vi "Create Execution Unit.vi"(8 "error in":errorcluster, 10 "Item Ref":T2=18446744073709551615 format="%.0x", 11 "Execution Unit Factory Implementation in":refnum<class "Execution Unit Factory.lvclass">) -> (0 "error out":errorcluster, 1 "Asynchronous Execution Units":T1[](array[typedef]) {"ReadWrite Channels" format="%.0x"; "Outgoing Channels" format="%.0x"; "Incoming Channels" format="%.0x"}, 2 "Inline Execution Units":T1[](array[typedef]) {"ReadWrite Channels" format="%.0x"; "Outgoing Channels" format="%.0x"; "Incoming Channels" format="%.0x"}, 3 "Execution Unit Factory Implementation out":refnum<class "Execution Unit Factory.lvclass">)   [LabVIEW 2020, in "Ballard ARINC 429 Engine.lvlib" / "Implementation.lvlib" / "Execution Unit Factory.lvclass"]
uses:
  Execution Unit Factory.lvclass
  <vilib>/NI VeriStand/Custom Device API/Custom Device Item Ref.ctl
  Interfaces/Controls/Execution Unit Information.ctl
  Interfaces/Execution Unit/Execution Unit.lvclass
  Rx Execution Unit/Rx Execution Unit.lvclass
  C:/Users/Administrator/Desktop/GIT/niveristand-ballard-arinc429-custom-device/Source/Custom Device Support/Engine/Interfaces/Execution Unit/Execution Unit.lvclass
  Tx Acyclic Labels Execution Unit/Tx Acyclic Labels Execution Unit.lvclass
  Tx Scheduled Labels Execution Unit/Tx Scheduled Labels Execution Unit.lvclass
  Execution Unit Factory.lvclass/Execution Unit Factory.ctl
  <vilib>/NI VeriStand/Custom Device API/Custom Device API.lvlib
  Interfaces/Interfaces.lvlib
  System Explorer/Implementation/Implementation.lvlib
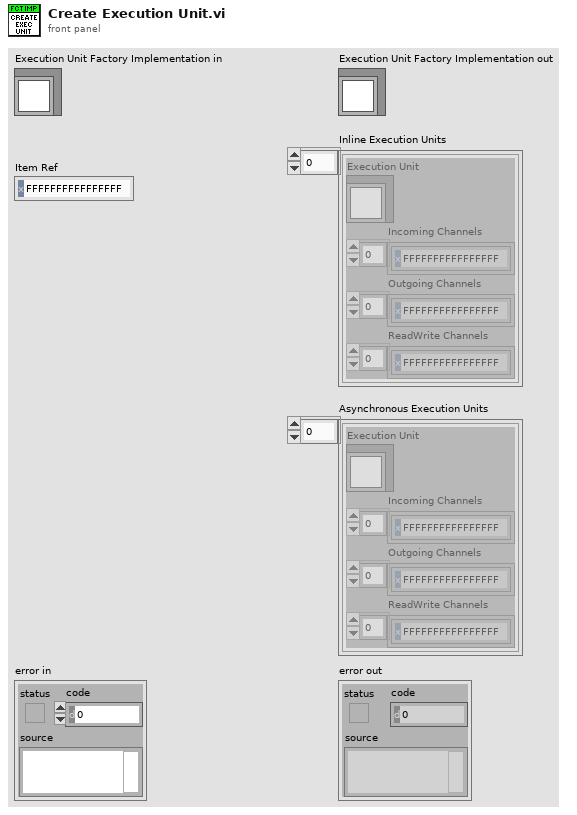
[diagram p1: front panel]
types:
  T1 = typedef "Ballard ARINC 429 Engine.lvlib/Interfaces.lvlib/Execution Unit Information.ctl" = cluster{"Execution Unit":refnum<class "Execution Unit.lvclass">, "Incoming Channels":T2[], "Outgoing Channels":T2[], "ReadWrite Channels":T2[]}
  T2 = typedef "Custom Device API.lvlib/Custom Device Item Ref.ctl" = u64
  T3 = typedef "Custom Device API.lvlib/Data Reference.ctl" = i32
  T4 = cluster{"receiving":T3, "specific errors":cluster{"gap":T3, "parity":T3, "long word ":T3, "bit timing":T3, "timeout":T3}}
  T5 = typedef "RT Hardware Channel Settings.ctl" = cluster{"channel #":u16, "channel handle":u64, "labels settings for RT":T6[]}
  T6 = typedef "RT Label Settings.ctl" = cluster{"Name":string, "xmlName":string, "label":T7, "transfer period":u32, "SDI_Enabled":bool, "SDI":u8, "parameter driver data":T8, "transfer type":T11, "has timestamp?":bool, "Label Disable/Trigger Channel Reference":T2, "Message Handle":u64, "Initialized?":bool, "Word Initial Raw Value":u32, "Label Timestamp Channel Data Reference":T3, "disabled":bool}
  T7 = typedef "Label.ctl" = u8
  T8 = typedef "RT Parameters.ctl" = cluster{"parameter definitions":T9[], "Tx parameter refs":T2[]}
  T9 = typedef "Parameter Definition.ctl" = cluster{"start index":i32, "size":i32, "encoding":T10, "signed":bool, "scale multiplier":dbl, "scale offset":dbl}
  T10 = typedef "Encoding and Decoding.lvlib/Encoding.ctl" = enum16{"BNR", "BCD", "Discrete"}
  T11 = typedef "Transfer Type.ctl" = enum16{"Scheduled", "Acyclic", "Block", "Strobe"}
  T12 = typedef "Custom Device API.lvlib/Custom Device Item Info.ctl" = cluster{"Name":string, "Is Channel":bool, "GUID":string, "Is Waveform":bool}
  T13 = cluster{"transfer type":T11, "Name":string, "hardware channel data":T5[], "Outgoing Channels":T2[], "ReadWrite Channels":T2[]}[]
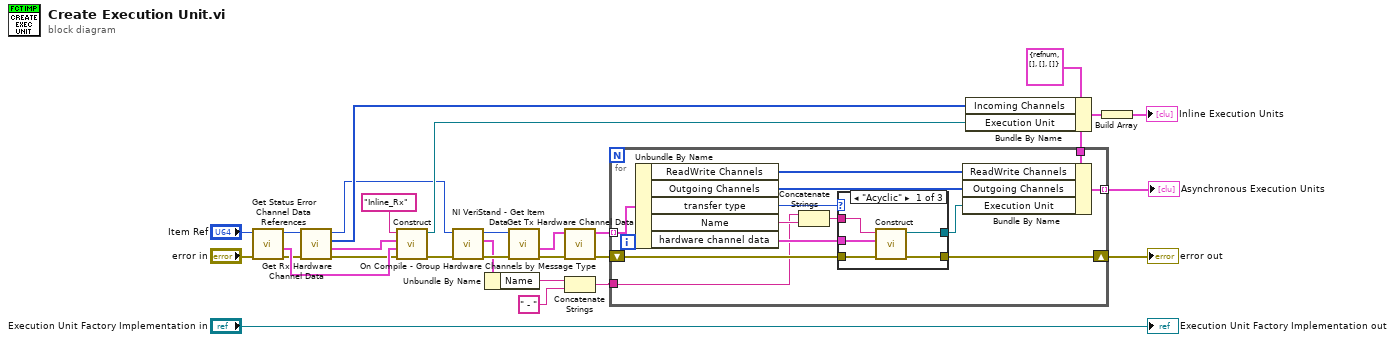
[diagram p0: block diagram]
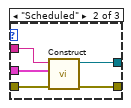
[diagram p2: hidden frame]
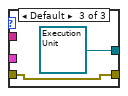
[diagram p3: hidden frame]
diagram:
  w10 = T1 {"Execution Unit"=refnum, "Incoming Channels"=[], "Outgoing Channels"=[], "ReadWrite Channels"=[]} ("Execution Unit Information")
  n1 = call "Get Status Error Channel Data References.vi"("error in"="error in", "custom device ref in"="Item Ref") -> ("error out"=w16:errorcluster, "status channel data references"=w20:T4, "custom device ref out"=w17:T2)  [unwired: 7 in]
  n2 = call "Get Rx Hardware Channel Data.vi"("error in"=w16, "custom device ref in"=w17) -> ("error out"=w15:errorcluster, "Rx hardware channel data"=w21:T5[], "incoming channels"=w25:T2[], "custom device ref out"=w7:T2)  [unwired: 6 in]
  n3 = call "Construct.vi"("error in"=w15, "status error channel data references"=w20, "RT hardware channels"=w21, "ID"="Inline_Rx") -> ("error out"=w8:errorcluster, "Ballard ARINC-429 Rx Execution Unit"=w14:refnum<class "Rx Execution Unit.lvclass">)  [unwired: 6 in]
  n4 = call <vilib>:"NI VeriStand - Get Item Data.vi"("error in (no error)"=w8, "Item Ref in"=w7) -> ("error out"=w5:errorcluster, "Item Info"=w4:T12, "Item Ref out"=w6:T2)  [unwired: 6 in, 1 out]
  n5 = Unbundle By Name(w4) -> ("Name"=w3:string)
  n6 = call "Get Tx Hardware Channel Data.vi"("error in"=w5, "custom device ref in"=w6) -> ("error out"=w23:errorcluster, "Tx hardware channel data"=w22:T5[])  [unwired: 6 in, 2 out]
  n7 = call "On Compile - Group Hardware Channels by Message Type.vi"("error in"=w23, "hardware channel data"=w22) -> ("error out"=w13:errorcluster, "hardware channel data by transfer type"=w11:T13)  [unwired: 8 in]
  n8 = Concatenate Strings(w3, " - " ("string")) -> (w1:string)
  n9 = for {
    shift-right: [w40] -> w12
    shift-left: w13 -> [w41]
    tunnel: w11 -> [w39] mode=indexing
    tunnel: w10 -> [w37]
    tunnel: [w35] -> w9 mode=indexing
    tunnel: w1 -> [w30]
    n10 = Unbundle By Name(w39) -> ("ReadWrite Channels"=w34:T2[], "Outgoing Channels"=w33:T2[], "transfer type"=w36:T11, "Name"=w31:string, "hardware channel data"=w32:T5[])
    n11 = Concatenate Strings(w30, w31) -> (w29:string)
    n12 = case shown="\"Acyclic\"" w36 {
      tunnel: w32 -> [w46 w51 _]
      tunnel: [w45 w50 refnum<class "Execution Unit.lvclass"> refnum ("Execution Unit")] -> w38
      tunnel: w41 -> [w44 w49 w52]
      tunnel: [w43 w48 w52] -> w40
      tunnel: w29 -> [w42 w47 _]
      frame "Acyclic" {
        n13 = call "Construct.vi"("error in"=w44, "RT hardware channels"=w46, "ID"=w42) -> ("error out"=w43:errorcluster, "Ballard ARINC-429 Tx Acyclic execution unit out"=w45:refnum<class "Tx Acyclic Labels Execution Unit.lvclass">)  [unwired: 7 in]
      }
      frame "Scheduled" {
        n14 = call "Construct.vi"("error in"=w49, "RT hardware channels"=w51, "ID"=w47) -> ("error out"=w48:errorcluster, "Ballard ARINC-429 Tx Execution Unit out"=w50:refnum<class "Tx Scheduled Labels Execution Unit.lvclass">)  [unwired: 7 in]
      }
      frame Default {
      }
    }
    n15 = Bundle By Name(cluster=w37, "ReadWrite Channels"=w34, "Outgoing Channels"=w33, "Execution Unit"=w38) -> (w35:T1)
  }
  "error out" <- w12
  "Asynchronous Execution Units" <- w9
  n16 = Bundle By Name(cluster=w10, "Incoming Channels"=w25, "Execution Unit"=w14) -> (w27:T1)
  n17 = Build Array(w27) -> (→"Inline Execution Units":T1[])
  "Execution Unit Factory Implementation out" <- "Execution Unit Factory Implementation in"
